vi "Destroy Mask.vi"(8 "error in (no error)":errorcluster, 11 "Rectangle Mask in":refnum<class "Rectangle Mask.lvclass">) -> (0 "error out":errorcluster)   [LabVIEW 2016, in "Rectangle Mask.lvclass"]
uses:
  Rectangle Mask.lvclass
  Panels.ctl
  Rectangle Mask.lvclass/Rectangle Mask.ctl
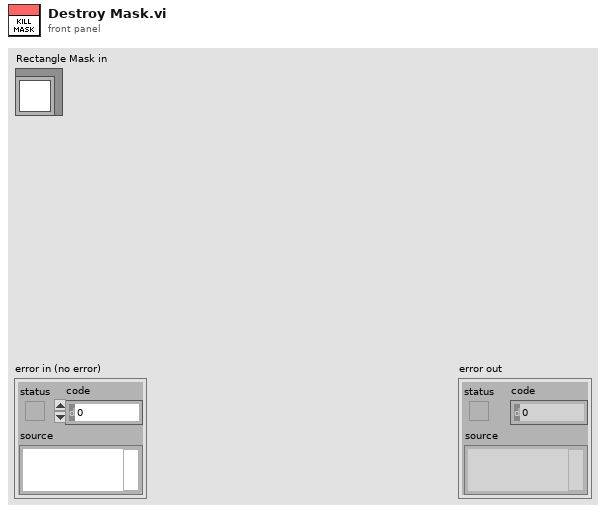
[diagram p1: front panel]
types:
  T1 = typedef "Rectangle Mask.lvclass/Panels.ctl" = cluster{"Left":refnum<vi>, "Top":refnum<vi>, "Right":refnum<vi>, "Bottom":refnum<vi>}
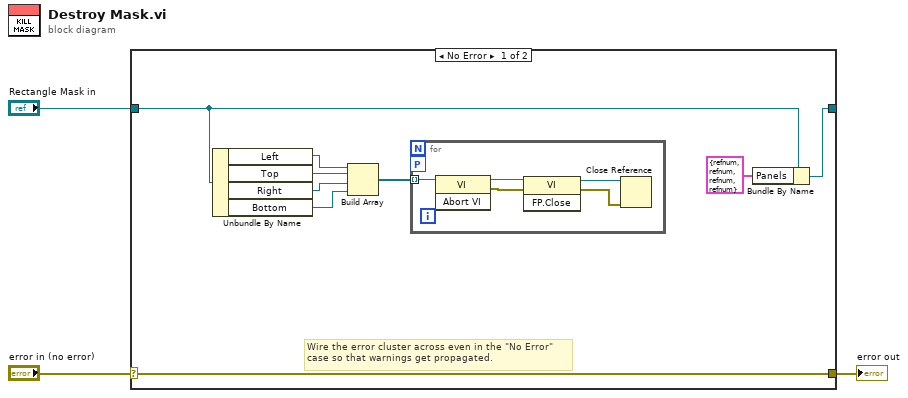
[diagram p0: block diagram]
diagram:
  n1 = case shown="No Error" "error in (no error)" {
    selector: "error in (no error)" -> [w12 w19]
    tunnel: [w12 w19] -> w2
    tunnel: [w4 w18] -> _
    tunnel: "Rectangle Mask in" -> [w6 w18]
    frame No Error {
      # "Wire the error cluster across even in the \"No Error\"\ncase so that warnings get propagated."
      n2 = Unbundle By Name(w6) -> ("Left"=w11:refnum<vi>, "Top"=w10:refnum<vi>, "Right"=w9:refnum<vi>, "Bottom"=w8:refnum<vi>)
      n3 = Build Array(w11, w10, w9, w8) -> (w7:refnum<vi>[])
      n4 = for {
        tunnel: w7 -> [w17] mode=indexing
        workers-P: _ -> [_]
        n5 = invoke class="VI" method="Abort VI"(reference=w17) -> (reference out=w14:refnum<vi>, error out=w16:errorcluster)  [unwired: 2 in, 1 out]
        n6 = invoke class="VI" method="FP.Close"(reference=w14, error in=w16) -> (reference out=w13:refnum<vi>, error out=w15:errorcluster)  [unwired: 1 in, 1 out]
        n7 = Close Reference(reference=w13, error in (no error)=w15) -> ()  [unwired: 1 out]
      }
      n8 = Bundle By Name(cluster=w6, "Panels"=T1 {"Left"=refnum, "Top"=refnum, "Right"=refnum, "Bottom"=refnum}) -> (w4:refnum<class "Rectangle Mask.lvclass">)
    }
    frame Error {
    }
  }
  "error out" <- w2
